vi "lab2.vi"() -> ()   [LabVIEW 2018]
panel:
  in  "stop":bool
  out "XOR":bool
  out "OR":bool
  out "AND":bool
  out "VOLTS IN":dbl
  in  "Numeric":dbl
  in  "switch \non/off 2":bool
  out "LED 3":bool
  out "LED 2":bool
  out "LED 1":bool
  in  "switch \non/off":bool
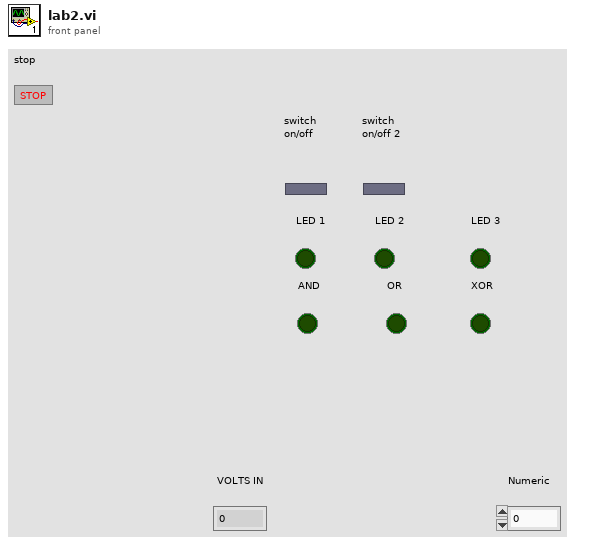
[diagram p1: front panel]
types:
  T1 = cluster{"data[0]":bool, "data[1]":bool, "data[2]":bool, "data[3]":bool, "data[4]":bool, "data[5]":bool, "data[6]":bool, "data[7]":bool, "data[8]":bool}
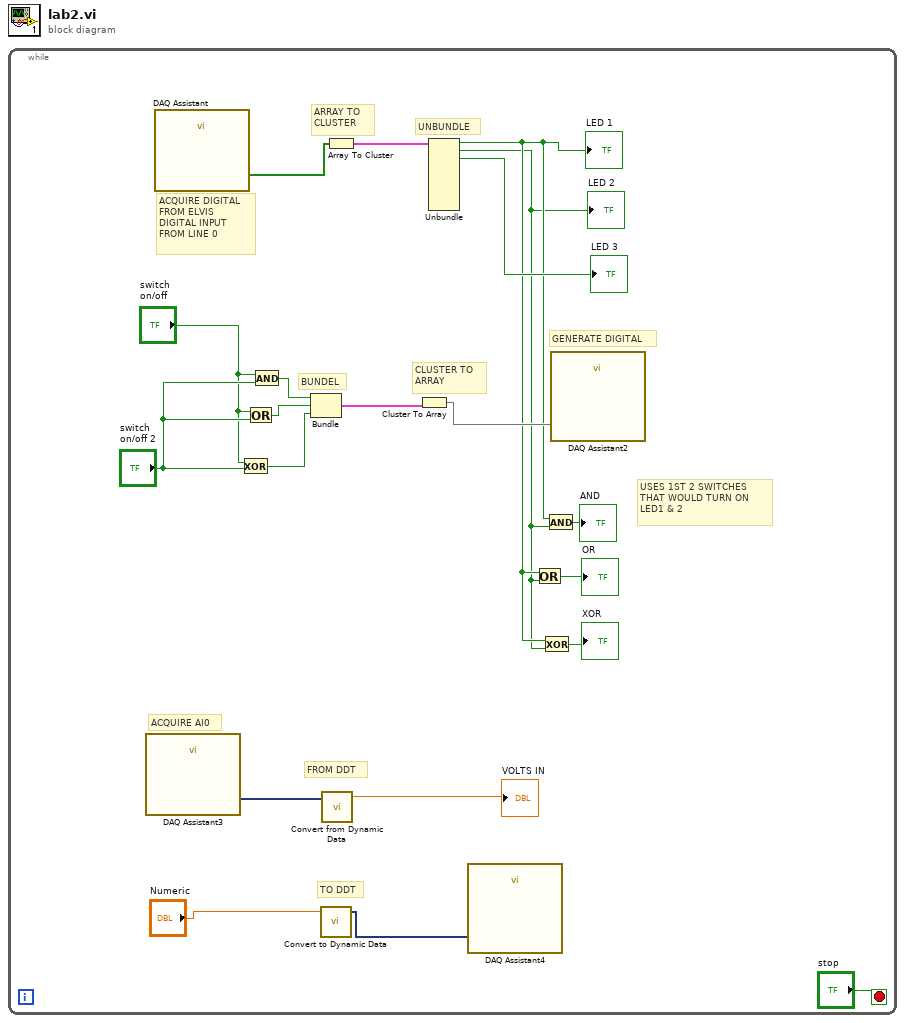
[diagram p0: block diagram]
diagram:
  n1 = while {
    stop <- "stop" stop-if-true
    # "USES 1ST 2 SWITCHES\nTHAT WOULD TURN ON\nLED1 & 2"
    # "TO DDT"
    # "FROM DDT"
    # "ACQUIRE AI0"
    # "GENERATE DIGITAL"
    # "CLUSTER TO \nARRAY"
    # "BUNDEL"
    # "UNBUNDLE"
    # "ARRAY TO \nCLUSTER"
    # "ACQUIRE DIGITAL\nFROM ELVIS \nDIGITAL INPUT\nFROM LINE 0"
    n2 = call "DAQ Assistant3"() -> ("data"=w16:dynamicdata)  [unwired: 17 in, 2 out]
    n3 = call "DAQ Assistant"() -> ("data"=w20:bool[])  [unwired: 17 in, 2 out]
    n4 = Exclusive Or(1:"switch \non/off 2", 2:"switch \non/off") -> (0:w6:bool)
    n5 = Or(x="switch \non/off", y="switch \non/off 2") -> (x .or. y?=w5:bool)
    n6 = And(x="switch \non/off", y="switch \non/off 2") -> (x .and. y?=w4:bool)
    n7 = Bundle(w4, w5, w6) -> (w7:cluster{bool, bool, bool})  [unwired: 1 in]
    n8 = call "Convert to Dynamic Data"("Double"="Numeric") -> ("Dynamic Data Type"=w13:dynamicdata)  [unwired: 3 in]
    n9 = call "Convert from Dynamic Data"("Dynamic Data Type"=w16) -> ("Scalar"=→"VOLTS IN":dbl)  [unwired: 3 in]
    n10 = Array To Cluster(array=w20) -> (cluster=w19:T1)
    n11 = Cluster To Array(cluster=w7) -> (array=w17:bool[])
    n12 = Unbundle(w19) -> ("data[0]"=w9:bool, "data[1]"=w8:bool, "data[2]"=→"LED 3":bool)  [unwired: 6 out]
    "LED 1" <- w9
    "LED 2" <- w8
    n13 = call "DAQ Assistant4"("data"=w13) -> ()  [unwired: 17 in, 2 out]
    n14 = Or(x=w9, y=w8) -> (x .or. y?=→"OR":bool)
    n15 = Exclusive Or(1:w8, 2:w9) -> (0:→"XOR":bool)
    n16 = And(x=w9, y=w8) -> (x .and. y?=→"AND":bool)
    n17 = call "DAQ Assistant2"("data"=w17) -> ()  [unwired: 17 in, 2 out]
  }
